vi "interpolate2D.vi"(10 "dimension":i32, 11 "MaxProj":u16[][](array[numeric])) -> (3 "Array":u16[][](array[numeric]))   [LabVIEW 2015]
panel:
  out "size(s)":i32[](array[numeric])
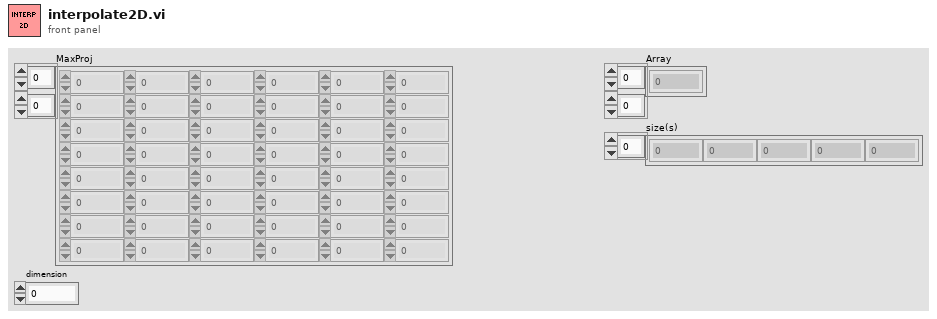
[diagram p1: front panel]
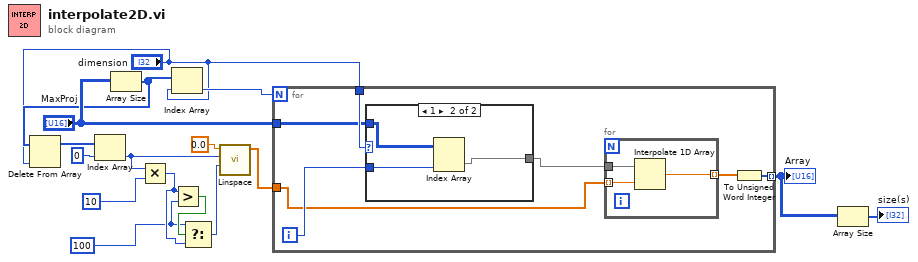
[diagram p0: block diagram]
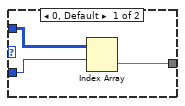
[diagram p2: hidden frame]
diagram:
  w1 = u16 100 ("y")
  n1 = Array Size(array="MaxProj") -> (size(s)=w13:i32[])
  n2 = Delete From Array(array=w13, index="dimension") -> (array with subset deleted=w11:i32[])  [unwired: 1 in, 1 out]
  n3 = Index Array(array=w11, index=0) -> (element=w9:i32)
  n4 = Multiply(x=w9, y=10) -> (x*y=w2:i32)
  n5 = Index Array(array=w13, index="dimension") -> (element=w16:i32)
  n6 = Greater?(x=w2, y=w1) -> (0:w4:bool)
  n7 = Select(t=w1, s=w4, f=w2) -> (s? t:f=w3:i32)
  n8 = call "Linspace.vi"("n"=w3, "End"=w9, "Start"=0.0) -> ("Array"=w7:dbl[])  [unwired: 8 in]
  n9 = for {
    N: w16 -> [_]
    tunnel: "MaxProj" -> [w22]
    tunnel: "dimension" -> [w23]
    tunnel: w7 -> [w19]
    tunnel: [w17] -> w6 mode=indexing
    i -> [w21]
    n10 = case shown="1" w23 {
      tunnel: w22 -> [w29 w32]
      tunnel: w21 -> [w28 w31]
      tunnel: [w27 w30] -> w20
      frame 0, Default {
        n11 = Index Array(array=w29, index (row)=w28) -> (element=w27:u16[])  [unwired: 1 in]
      }
      frame 1 {
        n12 = Index Array(array=w32, index (col)=w31) -> (element=w30:u16[])  [unwired: 1 in]
      }
    }
    n13 = for {
      tunnel: w20 -> [w26]
      tunnel: w19 -> [w25] mode=indexing
      tunnel: [w24] -> w18 mode=indexing
      n14 = Interpolate 1D Array(1:w25, 2:w26) -> (0:w24:dbl)
    }
    n15 = To Unsigned Word Integer(number=w18) -> (unsigned 16bit integer=w17:u16[])
  }
  "Array" <- w6
  n16 = Array Size(array=w6) -> (size(s)=→"size(s)":i32[])
